vi "Uv2_2022.vi"(1 "B(T)":dbl, 2 "Gamma0 humid air":dbl, 3 "xw":dbl, 4 "Temperature [K]":dbl) -> (0 "Uv2":dbl)   [LabVIEW 2016]
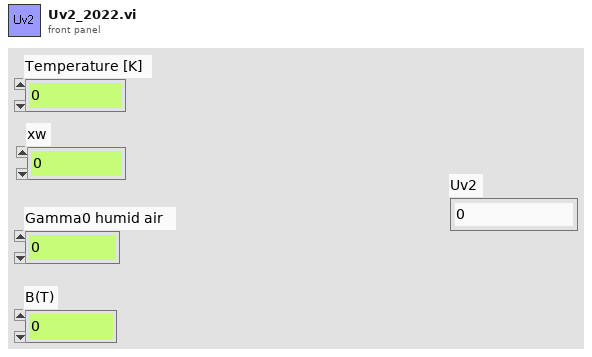
[diagram p1: front panel]
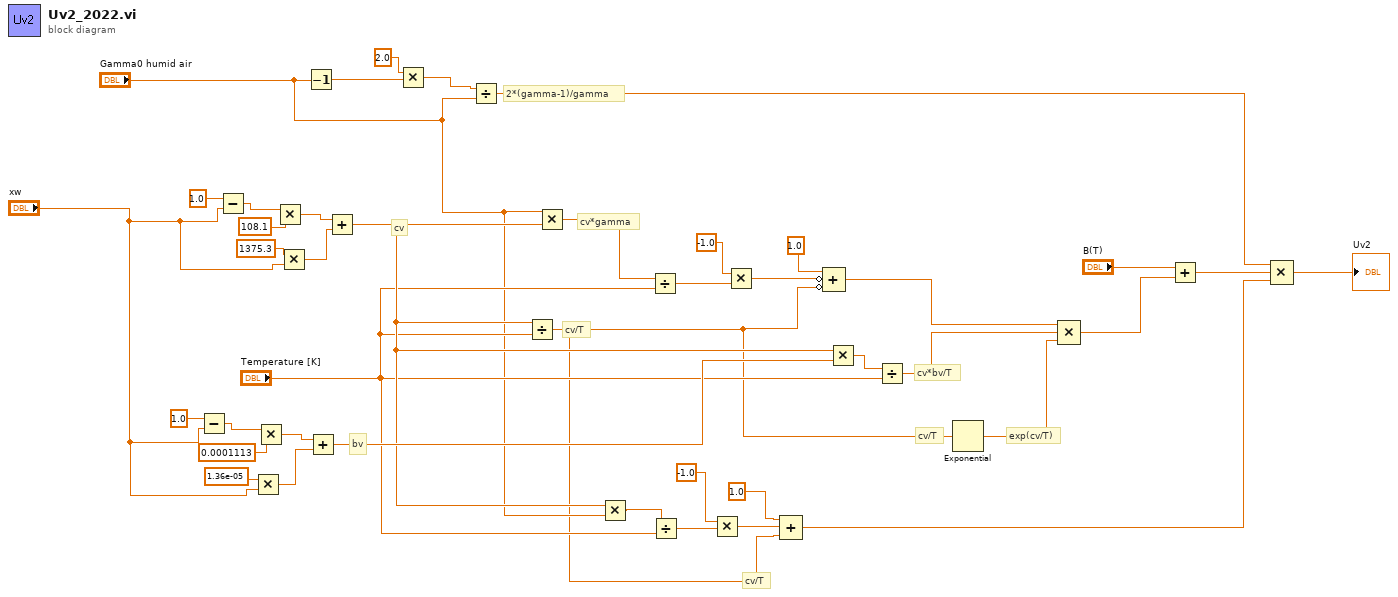
[diagram p0: block diagram]
diagram:
  # "cv*bv/T"
  # "exp(cv/T)"
  # "cv/T"
  # "cv/T"
  # "cv*gamma"
  # "cv/T"
  # "2*(gamma-1)/gamma"
  # "bv"
  # "cv"
  n1 = Subtract(x=1.0, y="xw") -> (x-y=w31:dbl)
  n2 = Subtract(x=1.0, y="xw") -> (x-y=w37:dbl)
  n3 = Multiply(x=1.36e-05, y="xw") -> (x*y=w27:dbl)
  n4 = Multiply(x=w31, y=0.0001113) -> (x*y=w29:dbl)
  n5 = Multiply(x=w37, y=108.1) -> (x*y=w35:dbl)
  n6 = Multiply(x=1375.3, y="xw") -> (x*y=w33:dbl)
  n7 = Decrement(x="Gamma0 humid air") -> (x-1=w2:dbl)
  n8 = Add(x=w29, y=w27) -> (x+y=w23:dbl)
  n9 = Add(x=w35, y=w33) -> (x+y=w11:dbl)
  n10 = Multiply(x=2.0, y=w2) -> (x*y=w40:dbl)
  n11 = Divide(x=w40, y="Gamma0 humid air") -> (x/y=w17:dbl)
  n12 = Divide(x=w11, y="Temperature [K]") -> (x/y=w1:dbl)
  n13 = Multiply(x="Gamma0 humid air", y=w11) -> (x*y=w25:dbl)
  n14 = Multiply(x=w11, y="Gamma0 humid air") -> (x*y=w15:dbl)
  n15 = Divide(x=w25, y="Temperature [K]") -> (x/y=w9:dbl)
  n16 = Divide(x=w15, y="Temperature [K]") -> (x/y=w5:dbl)
  n17 = Multiply(x=-1.0, y=w5) -> (x*y=w7:dbl)
  n18 = Multiply(x=-1.0, y=w9) -> (x*y=w10:dbl)
  n19 = Compound Arithmetic op=ADD(1.0, w7, w1) -> (w13:dbl)
  n20 = Compound Arithmetic op=ADD(1.0 ("x"), invert w10, invert w1) -> (w24:dbl)
  n21 = Multiply(x=w11, y=w23) -> (x*y=w22:dbl)
  n22 = Divide(x=w22, y="Temperature [K]") -> (x/y=w21:dbl)
  n23 = Exponential(1:w1) -> (0:w20:dbl)
  n24 = Compound Arithmetic op=MULTIPLY(w24, w21, w20) -> (w18:dbl)
  n25 = Add(x="B(T)", y=w18) -> (x+y=w16:dbl)
  n26 = Compound Arithmetic op=MULTIPLY(w17, w16, w13) -> (→"Uv2":dbl)
